vi "Do Core.vi"(8 "error in (no error)":errorcluster, 9 "Actor in":refnum<class "Actor.lvclass">, 11 "Reply Message":refnum<class "Read Parameters Msg.lvclass">) -> (0 "error out":errorcluster, 1 "Actor out":refnum<class "Actor.lvclass">, 2 "Reply":variant)   [LabVIEW 2015, in "Read Parameters Msg.lvclass"]
doc: "(<B>Filename</B>: Actor Framework.lvlib:Reply Msg.lvclass:Do Core.vi)\n\nDefines what an actor does when it receives <B>Reply Message</B>. This method also defines the <B>Reply</B> that is returned to the actor that sent <B>Reply Message</B>.\n\nBy default, this method does nothing, and <B>Reply</B> is the ancestor Message class. A child class must override this method to define behavior and specify a child of the Message class to return in the <B>Reply</B> output."
uses:
  Read Parameters Msg.lvclass
  <vilib>/ActorFramework/Actor/Actor.lvclass
  Mag Lab Measure Interface/Mag Lab Measure UI.lvclass
  Mag Lab Properties/Mag Lab Parameters.lvclass
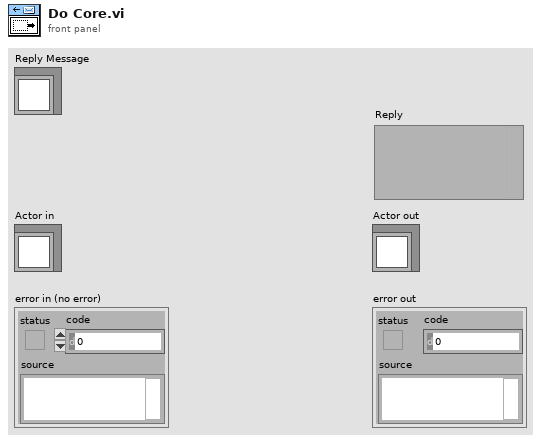
[diagram p1: front panel]
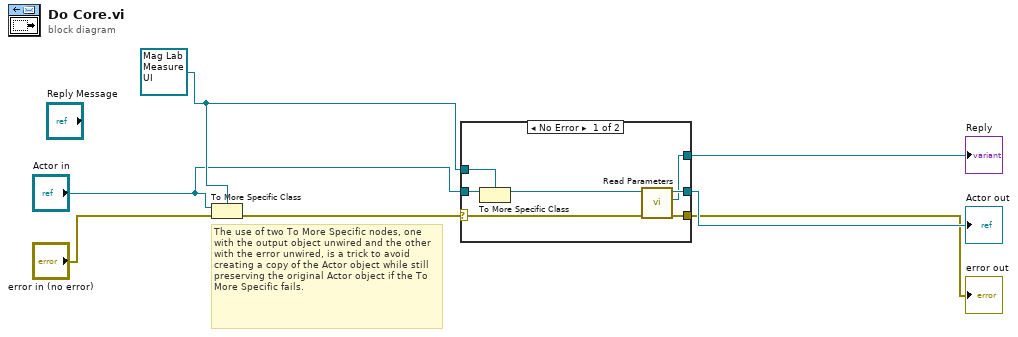
[diagram p0: block diagram]
diagram:
  w5 = refnum<class "Mag Lab Measure UI.lvclass"> refnum ("Actor in")
  # "The use of two To More Specific nodes, one with the output object unwired and the other with the error unwired, is a trick to avoid creating a copy of the Actor object while still preserving the original Actor object if the To More Specific fails."
  n1 = To More Specific Class(target class=w5, reference="Actor in", error in="error in (no error)") -> (error out=w7:errorcluster)  [unwired: 1 out]
  n2 = case shown="No Error" w7 {
    selector: w7 -> [w12 w16]
    tunnel: [w14 w16] -> w2
    tunnel: [w13 w15] -> w3
    tunnel: "Actor in" -> [w11 w15]
    tunnel: w5 -> [w10 _]
    tunnel: [w8 _] -> w1
    frame No Error {
      n3 = To More Specific Class(target class=w10, reference=w11) -> (specific class reference=w9:refnum<class "Mag Lab Measure UI.lvclass">)  [unwired: 1 in, 1 out]
      n4 = call-dynamic "Read Parameters.vi"("error in (no error)"=w12, "Mag Lab Root in"=w9) -> ("error out"=w14:errorcluster, "Mag Lab Parameters.lvclass"=w8:refnum<class "Mag Lab Parameters.lvclass">, "Mag Lab Root out"=w13:refnum<class "Mag Lab Measure UI.lvclass">)  [unwired: 7 in]
    }
    frame Error {
      # "If type check fails, pass the original object out again."
    }
  }
  "error out" <- w2
  "Actor out" <- w3
  "Reply" <- w1
